vi "String to Date.vi"(11 "Cal Due Date":string) -> (3 "time stamp":timestamp)   [LabVIEW 2010]
uses:
  <vilib>/Utility/miscctls.llb/LVDateTimeRec.ctl
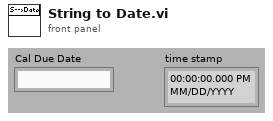
[diagram p1: front panel]
types:
  T1 = typedef "LVDateTimeRec.ctl" = cluster{"fractional second":dbl, "second":i32, "minute":i32, "hour":i32, "day of month":i32, "month":i32, "year":i32, "day of week":i32, "day of year":i32, "DST":i32}
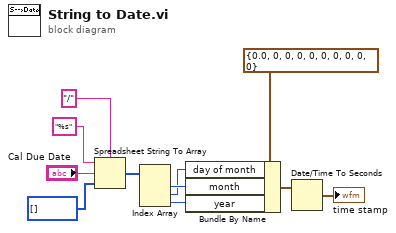
[diagram p0: block diagram]
diagram:
  n1 = Spreadsheet String To Array(delimiter (Tab)="/", format string="%s", spreadsheet string="Cal Due Date", array type (2D Dbl)=i32[] []) -> (array=w5:i32[])
  n2 = Index Array(array=w5) -> (element #1=w9:i32, element #2=w8:i32, element #3=w6:i32)  [unwired: 3 in]
  n3 = Bundle By Name(cluster=T1 {"fractional second"=0.0, "second"=0, "minute"=0, "hour"=0, "day of month"=0, "month"=0, "year"=0, "day of week"=0, "day of year"=0, "DST"=0} ("date time rec"), "day of month"=w8, "month"=w9, "year"=w6) -> (w7:T1)
  n4 = Date/Time To Seconds(2:w7) -> (0:→"time stamp":timestamp)  [unwired: 1 in]
